vi "thread_conductor.vi"(8 "entrée d'erreur (pas d'erreur)":errorcluster, 10 "Ce VI":refnum<vi>, 11 "File d'attente en entrée":refnum<queue>) -> (0 "sortie d'erreur":T5, 2 "File d'attente en sortie":refnum<queue>, 3 "Data Cluster":T1)   [LabVIEW 2020]
uses:
  support/Message Queue/Message Cluster.ctl
  controls/UI Data.ctl
  controls/Ctrl_Display.ctl
  controls/Ctrl_Ref.ctl
  support/Message Queue/All Message Queues.ctl
  controls/Ctrl_RefPad.ctl
  support/Message Queue/Enqueue Message (Single).vi
  <vilib>/Utility/error.llb/Error Cluster From Error Code.vi
  <vilib>/ErrorRing/Error Ring.xnode
  support/Message Queue/Message Queue.lvlib
  support/User Event - Stop/User Event - Stop.lvlib
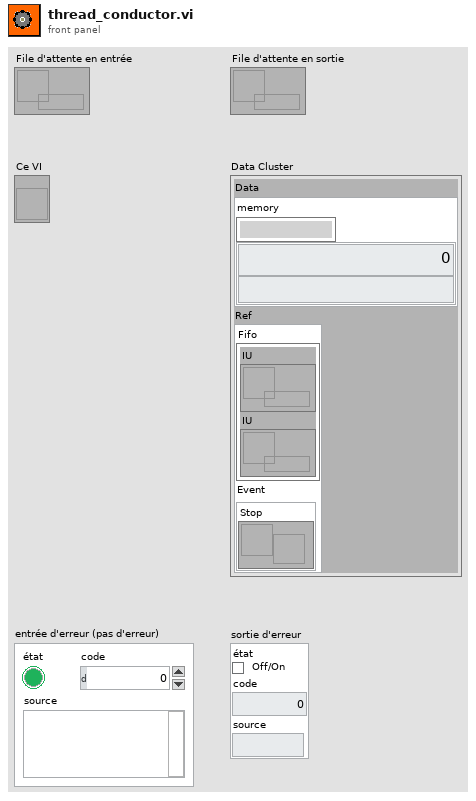
[diagram p1: front panel]
types:
  T1 = typedef "UI Data.ctl" = cluster{"Data":cluster{"memory":string, "Display":T2}, "Ref":T3}
  T2 = typedef "Ctrl_Display.ctl" = cluster{"Num":dbl, "Char":string}
  T3 = typedef "Ctrl_Ref.ctl" = cluster{"Fifo":T4, "Event":cluster{"Stop":refnum<user-event>}}
  T4 = typedef "Message Queue.lvlib/All Message Queues.ctl" = cluster{"Conductor":refnum<queue>, "IU":refnum<queue>}
  T5 = cluster{"état":bool, "code":i32, "source":string}
  T6 = typedef "Ctrl_RefPad.ctl" = cluster{"BTN_Ref":refnum<vi>, "CharPad":string}
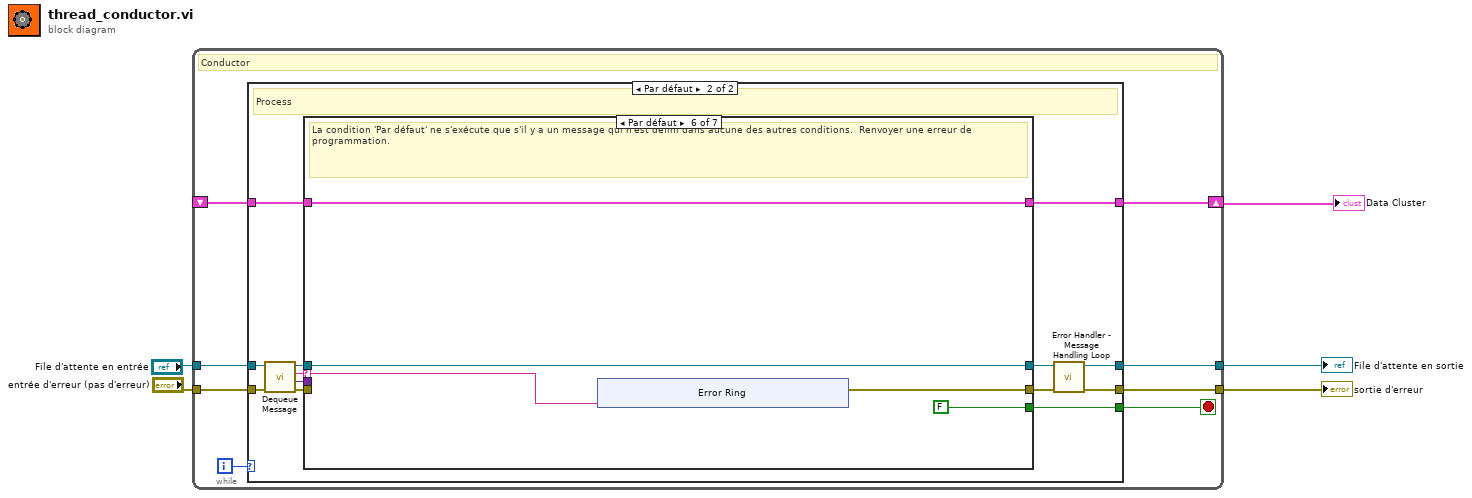
[diagram p0: block diagram]
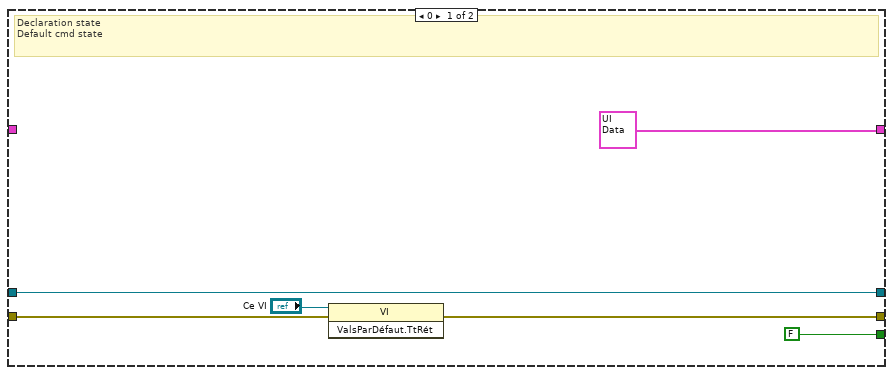
[diagram p2: hidden frame]
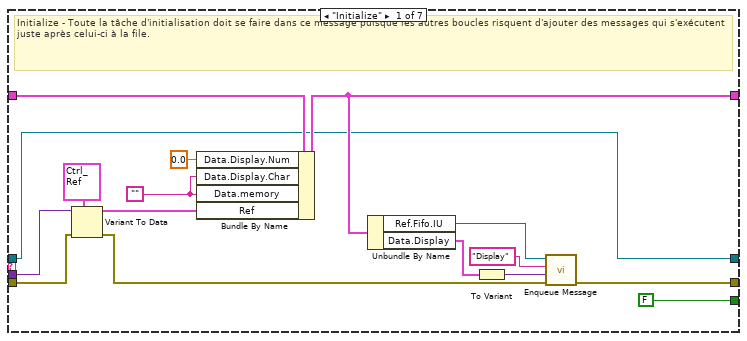
[diagram p3: hidden frame]
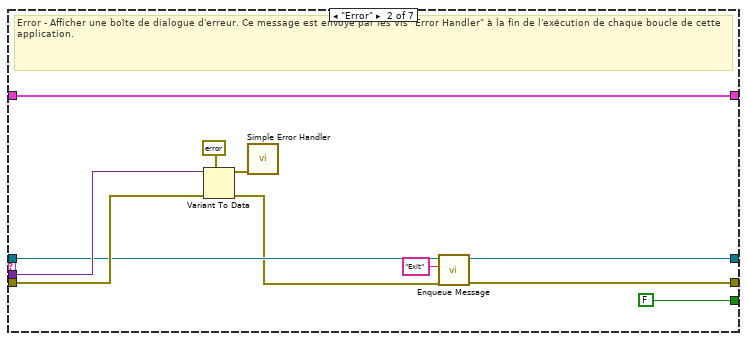
[diagram p4: hidden frame]
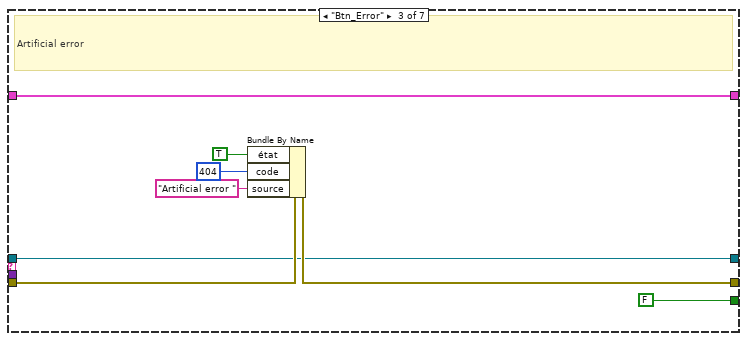
[diagram p5: hidden frame]
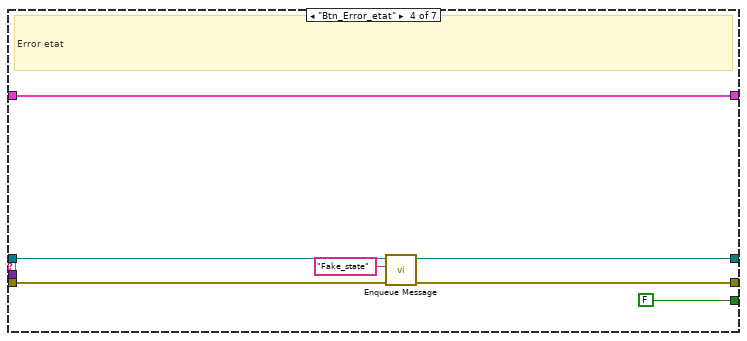
[diagram p6: hidden frame]
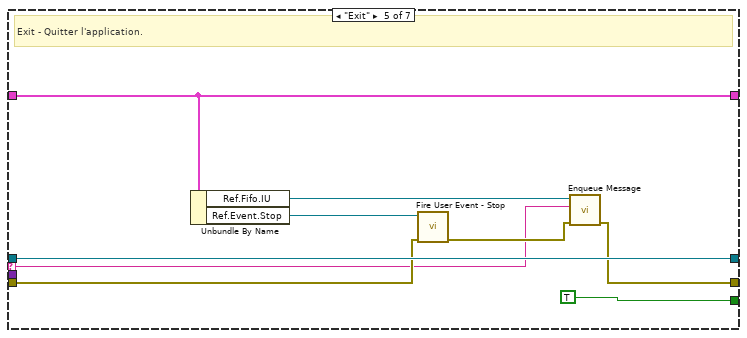
[diagram p7: hidden frame]
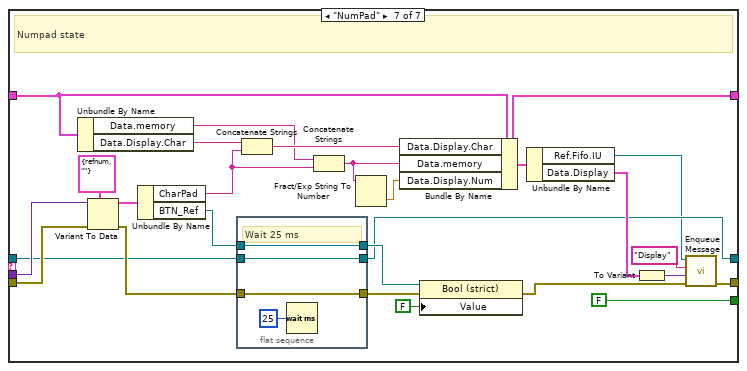
[diagram p8: hidden frame]
diagram:
  n1 = while {
    tunnel: "File d'attente en entrée" -> [w9]
    shift-right: [w12] -> w2
    shift-left: _ -> [w13]
    tunnel: "entrée d'erreur (pas d'erreur)" -> [w10]
    tunnel: [w8] -> w4
    tunnel: [w7] -> w3
    i -> [w6]
    stop <- w11 stop-if-true
    # "Conductor"
    n2 = case shown="Par défaut" w6 {
      tunnel: w13 -> [_ w32]
      tunnel: [T1 {"Data"={"memory"="", "Display"={"Num"=0.0, "Char"=""}}, "Ref"={"Fifo"={"Conductor"=refnum, "IU"=refnum}, "Event"={"Stop"=refnum}}} ("Data Cluster") w31] -> w12
      tunnel: [FALSE w30] -> w11
      tunnel: w10 -> [w15 w29]
      tunnel: w9 -> [w18 w25]
      tunnel: [w14 w23] -> w8
      tunnel: [w18 w20] -> w7
      frame 0 {
        # "Declaration state\nDefault cmd state"
        n3 = invoke class="VI" method="ValsParDéfaut.TtRét"(reference="Ce VI", error in=w15) -> (error out=w14:errorcluster)  [unwired: 1 in, 2 out]
      }
      frame Default {
        # "Process"
        n4 = call "Dequeue Message.vi"("error in (no error)"=w29, "File d'attente de messages"=w25) -> ("error out"=w28:T5, "Données de message"=w26:variant, "Message"=w27:string, "File d'attente de message dup."=w24:refnum<queue>)  [unwired: 6 in]
        n5 = case "Conditions des messages" shown="Par défaut" w27 {
          selector: w27 -> [_ _ _ _ w75 w86 _]
          tunnel: w24 -> [w35 w53 w61 w70 w80 w84 w105]
          tunnel: w28 -> [w45 w59 w67 w73 w79 _ w121]
          tunnel: [w48 w50 w65 w72 w77 w87 w117] -> w22
          tunnel: w32 -> [w47 w58 w66 w74 w82 w88 w116]
          tunnel: [w37 w58 w66 w74 w82 w88 w100] -> w31
          tunnel: [FALSE FALSE FALSE FALSE TRUE FALSE FALSE] -> w30
          tunnel: w26 -> [w44 w57 _ _ _ _ w120]
          tunnel: [w35 w52 w61 w71 w80 w84 w97] -> w21
          frame "Initialize" {
            w41 = ""
            # "Initialize - Toute la tâche d'initialisation doit se faire dans ce message puisque les autres boucles risquent d'ajouter des messages qui s'exécutent juste après celui-ci à la file."
            n6 = Variant To Data(error in=w45, type=T3 {"Fifo"={"Conductor"=refnum, "IU"=refnum}, "Event"={"Stop"=refnum}} ("Ref"), Variant=w44) -> (data=w38:T3, error out=w43:errorcluster)
            n7 = Bundle By Name(cluster=w47, "Data.Display.Num"=0.0, "Data.Display.Char"=w41, "Data.memory"=w41, "Ref"=w38) -> (w37:T1)
            n8 = Unbundle By Name(w37) -> ("Ref.Fifo.IU"=w36:refnum<queue>, "Data.Display"=w34:T2)
            n9 = To Variant(anything=w34) -> (Variant=w33:variant)
            n10 = call-poly "Enqueue Message.vi"("error in (no error)"=w43, "Données de message"=w33, "Message"="Display", "File d'attente de messages"=w36) -> ("error out"=w48:T5)  [unwired: 6 in, 1 out]
          }
          frame "Error" {
            # "Error - Afficher une boîte de dialogue d'erreur. Ce message est envoyé par les VIs \"Error Handler\" à la fin de l'exécution de chaque boucle de cette application."
            n11 = Variant To Data(error in=w59, type=errorcluster {"status"=FALSE, "code"=0, "source"=""} ("error constant"), Variant=w57) -> (data=w55:errorcluster, error out=w51:errorcluster)
            n12 = call <vilib>:"Simple Error Handler.vi"("error in (no error)"=w55) -> ()  [unwired: 4 in, 5 out]
            n13 = call-poly "Enqueue Message.vi"("error in (no error)"=w51, "Message"="Exit", "File d'attente de messages"=w53) -> ("error out"=w50:T5, "File d'attente de message dup."=w52:refnum<queue>)  [unwired: 7 in]
          }
          frame "Btn_Error" {
            # "Artificial error"
            n14 = Bundle By Name(cluster=w67, "état"=TRUE, "code"=404, "source"="Artificial error ") -> (w65:T5)
          }
          frame "Btn_Error_etat" {
            # "Error etat"
            n15 = call-poly "Enqueue Message.vi"("error in (no error)"=w73, "Message"="Fake_state", "File d'attente de messages"=w70) -> ("error out"=w72:T5, "File d'attente de message dup."=w71:refnum<queue>)  [unwired: 7 in]
          }
          frame "Exit" {
            # "Exit - Quitter l'application."
            n16 = Unbundle By Name(w82) -> ("Ref.Fifo.IU"=w76:refnum<queue>, "Ref.Event.Stop"=w81:refnum<user-event>)
            n17 = call "Fire User Event - Stop.vi"("error in (no error)"=w79, "Événement utilisateur - Arrêt"=w81) -> ("error out"=w78:T5)  [unwired: 9 in]
            n18 = call-poly "Enqueue Message.vi"("error in (no error)"=w78, "Message"=w75, "File d'attente de messages"=w76) -> ("error out"=w77:T5)  [unwired: 7 in, 1 out]
          }
          frame Default {
            # "La condition 'Par défaut' ne s'exécute que s'il y a un message qui n'est défini dans aucune des autres conditions.  Renvoyer une erreur de programmation."
            n19 = xnode ("Error Ring")("paramètre 0"=w86) -> ("sortie d'erreur"=w87:errorcluster)
          }
          frame "NumPad" {
            # "Numpad state"
            n20 = Unbundle By Name(w116) -> ("Data.memory"=w113:string, "Data.Display.Char"=w115:string)
            n21 = Variant To Data(error in=w121, type=T6 {"BTN_Ref"=refnum, "CharPad"=""} ("cluster"), Variant=w120) -> (data=w109:T6, error out=w106:errorcluster)
            n22 = Unbundle By Name(w109) -> ("CharPad"=w108:string, "BTN_Ref"=w107:refnum<vi>)
            n23 = flat-sequence {
              tunnel: w107 -> [w124]
              tunnel: [w124] -> w103
              tunnel: w106 -> [w123]
              tunnel: w105 -> [w122]
              tunnel: [w123] -> w104
              tunnel: [w122] -> w97
              frame #0 {
                # "Wait 25 ms"
                n24 = Wait (ms)(milliseconds to wait=u32 25 ("attente (ms)")) -> ()  [unwired: 1 out]
              }
            }
            n25 = Concatenate Strings(w115, w108) -> (w114:string)
            n26 = Concatenate Strings(w113, w108) -> (w112:string)
            n27 = Fract/Exp String To Number(string=w112) -> (number=w111:dbl)  [unwired: 3 in, 1 out]
            n28 = Bundle By Name(cluster=w116, "Data.Display.Char"=w114, "Data.memory"=w112, "Data.Display.Num"=w111) -> (w100:T1)
            n29 = property class="Bool (strict)"(reference=w103, error in=w104, "Value"=FALSE ("Valeur")) -> (error out=w102:errorcluster)  [unwired: 1 out]
            n30 = Unbundle By Name(w100) -> ("Ref.Fifo.IU"=w96:refnum<queue>, "Data.Display"=w99:T2)
            n31 = To Variant(anything=w99) -> (Variant=w98:variant)
            n32 = call-poly "Enqueue Message.vi"("error in (no error)"=w102, "Données de message"=w98, "Message"="Display", "File d'attente de messages"=w96) -> ("error out"=w117:T5)  [unwired: 6 in, 1 out]
          }
        }
        n33 = call "Error Handler - Message Handling Loop.vi"("error in (no error)"=w22, "File d'attente de messages"=w21) -> ("erreur en entrée dup."=w23:T5, "File d'attente de message dup."=w20:refnum<queue>)  [unwired: 8 in]
      }
    }
  }
  "sortie d'erreur" <- w4
  "File d'attente en sortie" <- w3
  "Data Cluster" <- w2
